vi "Check for Messages.vi"(0 "Array":refnum<class "Network Command Processor.lvclass">[](array[class])) -> (14 "Boolean":bool)   [LabVIEW 2014, in "Controller.lvlib" / "Controller.lvclass"]
uses:
  Controller.lvclass
  Message Handlers/Network Command Processor.lvclass
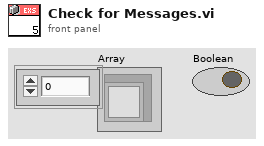
[diagram p1: front panel]
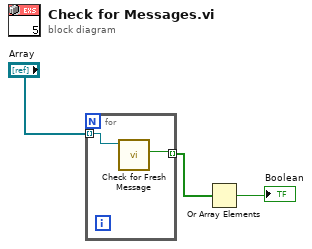
[diagram p0: block diagram]
diagram:
  n1 = for {
    tunnel: "Array" -> [w5] mode=indexing
    tunnel: [w4] -> w2 mode=indexing
    n2 = call-dynamic "Check for Fresh Message.vi"("Network Command Processor in"=w5) -> ("Enqueuer not Valid"=w4:bool)  [unwired: 7 in, 3 out]
  }
  n3 = Or Array Elements(Boolean array=w2) -> (logical OR=→"Boolean":bool)
